vi "DropVI_MQTT Server_Tracing.vi"() -> ()   [LabVIEW 2013]
uses:
  PacketTracer/PacketTracer.lvclass
  <vilib>/LabVIEW Open Source Project/Connection/Connection/Connection.lvclass
  Server class/Server.lvclass/Server.ctl
  <vilib>/LabVIEW Open Source Project/MQTT Connection/MQTT_Base/Base Class/MQTT_Base.lvclass/MQTT_Base.ctl
  <vilib>/LabVIEW Open Source Project/MQTT Control Packets/Control Packets/PUBLISH/PUBLISH.lvclass
  Server class/Server.lvclass
  <vilib>/LabVIEW Open Source Project/MQTT Connection/MQTT_Base/Base Class/MQTT_Base.lvclass
  <vilib>/LabVIEW Open Source Project/MQTT Control Packets/Control Packets/ControlPacket/ControlPacket.lvclass
  <vilib>/LabVIEW Open Source Project/Connection/Connection.TCP/Connection.TCP.lvclass
panel:
  out "Inbound Message":string
  out "error server":errorcluster
  out "NbConnections":u32
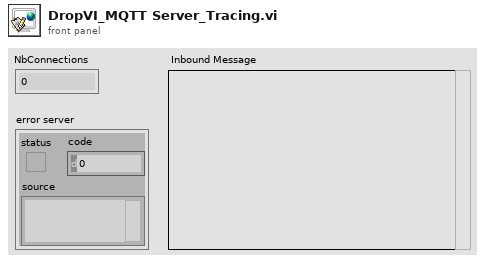
[diagram p1: front panel]
types:
  T1 = typedef "MQTT Base.lvlib/MQTT_Base.lvclass/Public Events -- cluster.ctl" = cluster{"Stop Event":refnum<user-event>, "Error Event":refnum<user-event>, "Inbound Message":refnum<user-event>}
  T2 = typedef "MQTT Server.lvlib/Server.lvclass/Public Events -- cluster.ctl" = cluster{"NbConnections":refnum<user-event>, "Client Event":refnum<user-event>}
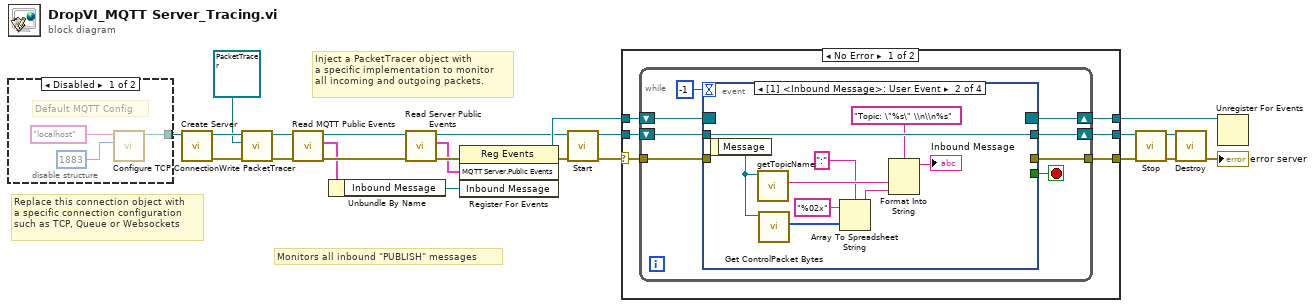
[diagram p0: block diagram]
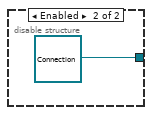
[diagram p2: hidden frame]
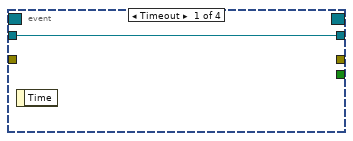
[diagram p3: hidden frame]
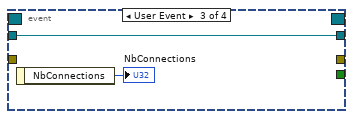
[diagram p4: hidden frame]
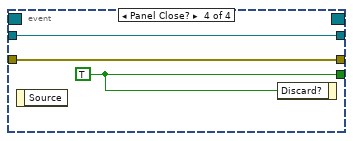
[diagram p5: hidden frame]
diagram:
  # "Replace this connection object with\na specific connection configuration\nsuch as TCP, Queue or Websockets"
  # "Inject a PacketTracer object with\na specific implementation to monitor\nall incoming and outgoing packets."
  # "Monitors all inbound \"PUBLISH\" messages"
  n1 = disable-structure shown="Disabled" {
    disable-tunnel: [w26 refnum<class "Connection.lvclass"> refnum ("Connection Configuration")] -> w1
    frame Disabled {
      # "Default MQTT Config"
      n2 = call <vilib>:"Configure TCP Connection.vi"("remote port (80)"=u16 1883, "address (localhost)"="localhost") -> ("Connection.TCP"=w26:refnum<class "Connection.TCP.lvclass">)  [unwired: 8 in, 1 out]
    }
    frame Enabled {
    }
  }
  n3 = call "Create Server.vi"("Connection Configuration"=w1) -> ("error out"=w4:errorcluster, "Server"=w6:refnum<class "Server.lvclass">)  [unwired: 9 in]
  n4 = call "Write PacketTracer.vi"("error in (no error)"=w4, "PacketTracer"=refnum<class "PacketTracer.lvclass"> refnum ("MQTT Server.lvlib:PacketTracer.lvclass"), "Server in"=w6) -> ("error out"=w3:errorcluster, "Server out"=w5:refnum<class "Server.lvclass">)  [unwired: 7 in]
  n5 = call <vilib>:"Read MQTT Public Events.vi"("error in (no error)"=w3, "MQTT_Base in"=w5) -> ("error out"=w9:errorcluster, "MQTT Public Events"=w8:T1, "MQTT_Base out"=w10:refnum<class "Server.lvclass">)  [unwired: 7 in]
  n6 = Unbundle By Name(w8) -> ("Inbound Message"=w7:refnum<user-event>)
  n7 = call "Read Server Public Events.vi"("error in (no error)"=w9, "Server in"=w10) -> ("error out"=w23:errorcluster, "MQTT Server.Public Events"=w22:T2, "Server out"=w19:refnum<class "Server.lvclass">)  [unwired: 7 in]
  n8 = register-events(error in=w23, w22, w7) -> (reference out=w21:refnum<event-registration>, error out=w17:errorcluster)  [unwired: 1 in]
  n9 = call <vilib>:"Start.vi"("error in (no error)"=w17, "MQTT_Base in"=w19) -> ("error out"=w16:errorcluster, "MQTT_Base out"=w18:refnum<class "Server.lvclass">)  [unwired: 7 in, 1 out]
  n10 = case shown="No Error" w16 {
    selector: w16 -> [w28 w57]
    tunnel: w18 -> [w33 w59]
    tunnel: [w32 w59] -> w13
    tunnel: w21 -> [w31 w58]
    tunnel: [w30 w58] -> w20
    tunnel: [w29 w57] -> w11
    frame No Error {
      n11 = while {
        shift-right: [w38] -> w32
        shift-left: w33 -> [w40]
        tunnel: [w35] -> w29
        tunnel: w28 -> [w34]
        shift-right: [w36] -> w30
        shift-left: w31 -> [w37]
        stop <- w39 stop-if-true
        n12 = event shown="[1] <Inbound Message>: User Event" {
          selector: w37 -> [_ _ _ _]
          dyn-events: [_ _ _ _] -> w36
          timeout: -1 -> [_ _ _ _]
          tunnel: w40 -> [w42 w51 w53 w56]
          tunnel: [_ _ _ w54] -> w39
          tunnel: [w42 w51 w53 w56] -> w38
          tunnel: [_ _ _ w55] -> w35
          tunnel: w34 -> [_ _ _ w55]
          event Timeout {
            n13 = event-data() -> ()  [unwired: 1 in, 1 out]
          }
          event User Event {
            n14 = event-data() -> ("Message"=w50:refnum<class "PUBLISH.lvclass">)  [unwired: 1 in]
            n15 = call <vilib>:"getTopicName.vi"("PUBLISH in"=w50) -> ("Topic"=w49:string)  [unwired: 8 in, 2 out]
            n16 = call <vilib>:"Get ControlPacket Bytes.vi"("ControlPacket"=w50) -> ("Bytes Stream"=w46:u8[])  [unwired: 7 in, 3 out]
            n17 = Array To Spreadsheet String(delimiter (Tab)=":", array=w46, 3:"%02x" ("format string")) -> (spreadsheet string=w43:string)
            n18 = Format Into String(format string="Topic: \"%s\" \\n\\n%s", w49, w43) -> (resulting string=→"Inbound Message":string)  [unwired: 2 in, 1 out]
          }
          event User Event {
            n19 = event-data() -> ("NbConnections"=→"NbConnections":u32)  [unwired: 1 in]
          }
          event Panel Close? {
            w54 = TRUE ("Discard?")
            n20 = event-data() -> ()  [unwired: 1 in, 1 out]
            n21 = event-data("Discard?"=w54) -> ()  [unwired: 1 in, 1 out]
          }
        }
      }
    }
    frame Error {
    }
  }
  n22 = call <vilib>:"Stop.vi"("error in (no error)"=w11, "MQTT_Base in"=w13) -> ("error out"=w12:errorcluster, "MQTT_Base out"=w14:refnum<class "Server.lvclass">)  [unwired: 7 in, 1 out]
  n23 = call <vilib>:"Destroy.vi"("error in (no error)"=w12, "MQTT_Base in"=w14) -> ("error out"=→"error server":errorcluster)  [unwired: 8 in, 1 out]
  n24 = Unregister For Events(event registration refnum=w20) -> ()  [unwired: 1 in, 1 out]
